vi "New Session Prompt (Non Actor).vi"(8 "error in (no error)":errorcluster, 11 "VISA resource name":refnum<visa-resource-name>) -> (0 "error out":errorcluster, 1 "Time Cluster":cluster{"Warm-Up":dbl, "Measure":dbl}, 2 "Continuous?":bool, 3 "VISA resource name out":refnum<visa-resource-name>, 4 "Array 2":T1[](array[typedef]) {"Thermocouple Type (0: J) 2" items=["J", "K", "E", "T", "N", "R", "S", "B", "C"]; "Channel" min=0 max=20 step=1; "Function (5: Temp)" items=["OFF", "TEMP"]})   [LabVIEW 2013, in "Generic Data Logger.lvlib" / "Fluke 2625A (Hydra II).lvlib" / "Fluke 2625A (Hydra II).lvclass"]
uses:
  Fluke 2625A (Hydra II).lvclass
  Unit Measurement.ctl
  <instrlib>/Fluke 2625A/Fluke 2625A.lvlib
panel:
  in  "Measurement":enum32{"Continuous", "Timed"}(radio)
  out "Array of channels out":bool[](array[boolean])
  in  "Array":T1[](array[typedef]) {"Thermocouple Type (0: J) 2" items=["J", "K", "E", "T", "N", "R", "S", "B", "C"]; "Channel" min=0 max=20 step=1; "Function (5: Temp)" items=["OFF", "VDC", "VAC", "OHMS", "FREQ", "TEMP"]}
  in  "Stop Button":bool
  in  "Temp Scale":u16(ring)=1 items=["C", "F"]
  in  "Measure":dbl format="%<%H:%M:%S>t"
  in  "Warm-Up":dbl format="%<%H:%M:%S>t"
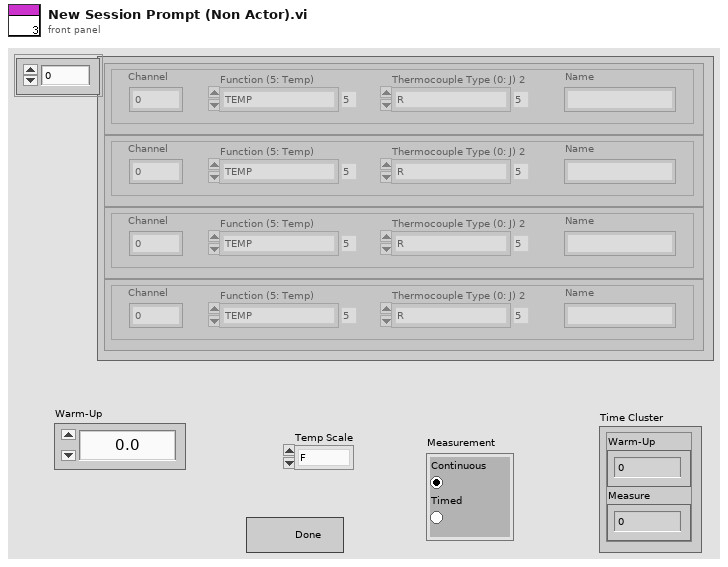
[diagram p1: front panel]
types:
  T1 = typedef "Unit Measurement.ctl" = cluster{"Function (5: Temp)":u16, "Channel":i8, "Thermocouple Type (0: J) 2":u16, "Name":string}
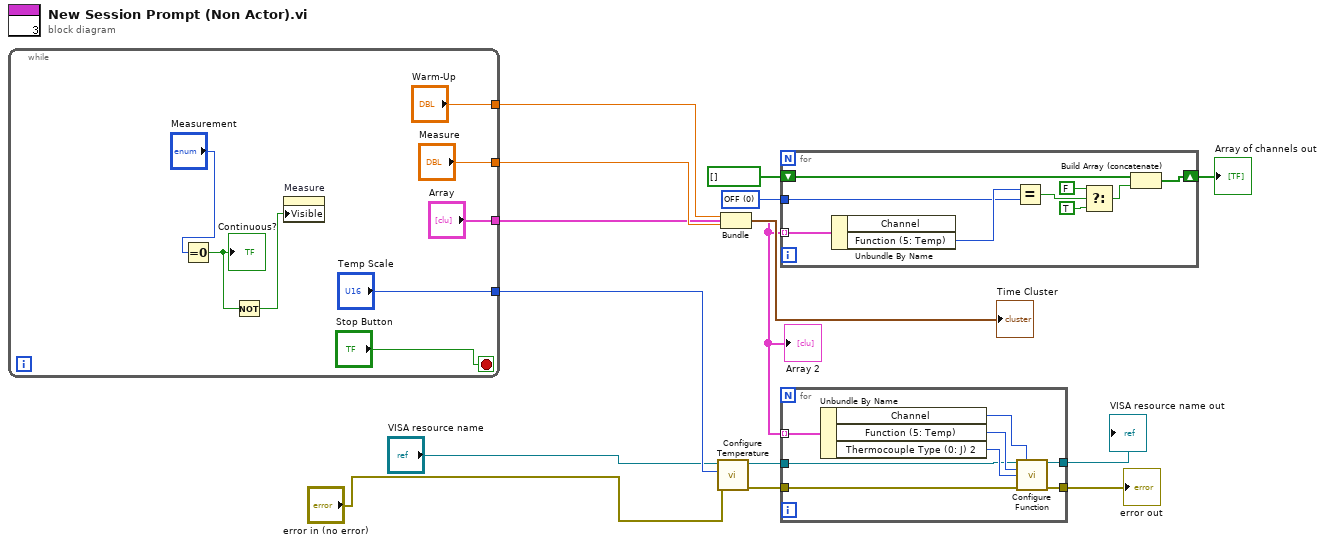
[diagram p0: block diagram]
diagram:
  w5 = u16 0 items=["OFF", "TEMP"] ("Function (5: Temp)")
  n1 = while {
    tunnel: ["Array"] -> w7
    tunnel: ["Temp Scale"] -> w11
    tunnel: ["Measure"] -> w10
    tunnel: ["Warm-Up"] -> w9
    stop <- "Stop Button" stop-if-true
    n2 = Equal To 0?(x="Measurement") -> (x = 0?=w17:bool)
    "Continuous?" <- w17
    n3 = Not(x=w17) -> (.not. x?=w15:bool)
    n4 = property on="Measure" class="DigNum (strict)"("Visible"=w15) -> ()  [unwired: 2 in, 2 out]
  }
  "Array 2" <- w7
  n5 = call <instrlib>:"Configure Temperature.vi"("error in (no error)"="error in (no error)", "Temp Scale"=w11, "VISA resource name"="VISA resource name") -> ("error out"=w13:errorcluster, "VISA resource name out"=w14:refnum<visa-resource-name>)  [unwired: 6 in, 1 out]
  n6 = Bundle("Warm-Up"=w9, "Measure"=w10) -> (→"Time Cluster":cluster{"Warm-Up":dbl, "Measure":dbl})  [unwired: 1 in]
  n7 = for {
    tunnel: w7 -> [w31] mode=indexing
    shift-right: [w27] -> w4
    shift-left: bool[] [] ("Array of channels in") -> [w28]
    tunnel: w5 -> [w29]
    n8 = Unbundle By Name(w31) -> ("Function (5: Temp)"=w30:u16)  [unwired: 1 out]
    n9 = Equal?(x=w30, y=w29) -> (x = y?=w26:bool)
    n10 = Select(t=FALSE, s=w26, f=TRUE) -> (s? t:f=w23:bool)
    n11 = Build Array (concatenate)(w28, w23) -> (w27:bool[])
  }
  "Array of channels out" <- w4
  n12 = for {
    tunnel: w7 -> [w39] mode=indexing
    tunnel: w14 -> [w33]
    tunnel: w13 -> [w35]
    tunnel: [w34] -> w12
    tunnel: [w32] -> w3
    n13 = Unbundle By Name(w39) -> ("Channel"=w36:i8, "Function (5: Temp)"=w38:u16, "Thermocouple Type (0: J) 2"=w37:u16)
    n14 = call <instrlib>:"Configure Function.vi"("VISA resource name"=w33, "Channel"=w36, "Function (5: Temp)"=w38, "Thermocouple Type (0: J) 2"=w37, "error in (no error)"=w35) -> ("VISA resource name out"=w32:refnum<visa-resource-name>, "error out"=w34:errorcluster)  [unwired: 7 in, 2 out]
  }
  "error out" <- w12
  "VISA resource name out" <- w3
